vi "Heart Sound TFA.vi"() -> ()   [LabVIEW 2023]
doc: "This example shows the application of the Time Frequency Analysis VIs in heart sound signal processing. \n\nTime frequency analysis has been widely applied in heart sound signal processing. You can use the Time Frequency Spectrogram Express VI to perform different methods for time-frequency representations. The frequency modulation of heart sound signals can be investigated easily in the time-frequency domain.\n\nThis example uses the Time Frequency Spectrogram Express VI to compute the adaptive spectrogram of the heart sound signal and uses the TFA Adaptive Transform VI to detect the modulation parameters of the heart sound signal.\n\n<b>Instructions:</b>\n1) Run this VI.\n2) Observe the <b>Spectrogram of Heart Sound</b> and the values of the detected chirplets in the <b>Chirplet Info</b> to learn the frequency modulation of heart sound."
uses:
  <vilib>/addons/Time Frequency Analysis/typedefs.llb/TFA Data.ctl
  Instance           5 23Saved   Heart Sound TFA .vi
  <vilib>/addons/Time Frequency Analysis/Transform.llb/TFA Adaptive Transform (Waveform).vi
  <vilib>/addons/Time Frequency Analysis/_control.llb/TFA Configure Spectrogram Indicator (Predefined Color Table).vi
  <vilib>/addons/_Advanced Signal Processing/NI_AdvSigProcTFA.lvlib
panel:
  out "aspt-left-top":bool
  out "Chirplet info":T1(array[cluster]) {"chirp rate" format="%#_2p Hz/s"; "frequency" format="%#_2p Hz"; "center" format="%#_2ps"; "standard deviation" format="%#_2ps"; "amplitude" format="%.2p"}
  out "Spectrogram of Heart Sound":dbl[][](graph)
  out "Heart Sound":waveform(dbl)(graph)
  # "Overview: Shows the application of the Time Frequency Analysis VIs in heart sound signal processing.\nRequirements: LabVIEW Full Development System, Advanced Signal Processing Toolkit\nInstructions: \n1. Run this VI.\n2. Observe the Spectrogram of Heart Sound and the values of the detected chirplets in the Chirplet Info to learn the frequency modulation of heart sound."
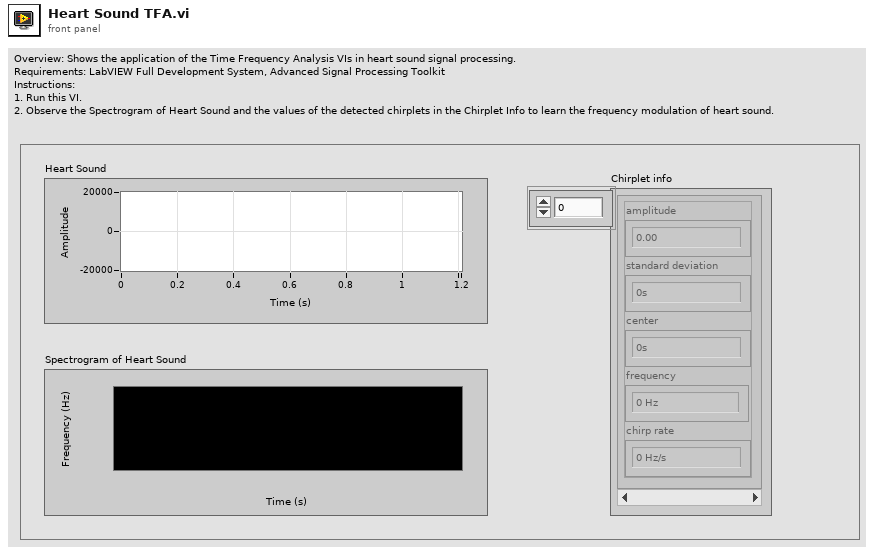
[diagram p1: front panel]
types:
  T1 = cluster{"amplitude":cdb, "standard deviation":dbl, "center":dbl, "frequency":dbl, "chirp rate":dbl}[]
  T2 = typedef "NI_AdvSigProcTFA.lvlib/TFA Data.ctl" = u16
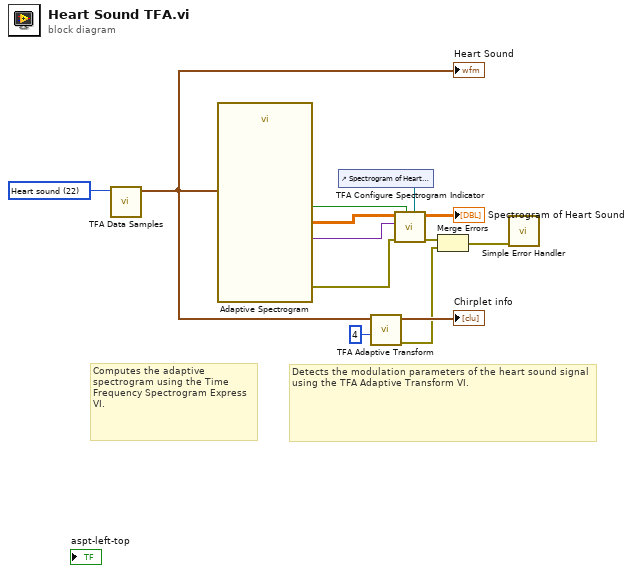
[diagram p0: block diagram]
diagram:
  w5 = T2 22 items=["PC Fan"=0, "Noisy Chirps"=1, "TDR 1"=2, "TDR 2"=3, "Liquefaction"=4, "Liquefaction Free"=5, "Aneurysm"=6, "Bat"=7, "RF"=8, "Two Gaussian"=9, "Three Gaussian"=10, "Chirp"=11, "Gaussian Chirp"=12, "Cross Chirp"=13, "Doppler"=14, "HOP"=15, "TF Sine"=16, "Three Tone"=17, "Four Tone"=23, "Blood Flow Doppler (phase a)"=20, "Blood Flow Doppler (phase b)"=21, "Heart sound"=22, "-"=18, "Random Noise"=19] ("data")
  # "Detects the modulation parameters of the heart sound signal using the TFA Adaptive Transform VI."
  # "Computes the adaptive spectrogram using the Time Frequency Spectrogram Express VI."
  n1 = call <vilib>:"TFA Data Samples.vi"("data"=w5) -> ("signal"=w6:waveform(dbl))  [unwired: 10 out]
  "Heart Sound" <- w6
  n2 = call "Adaptive Spectrogram"("Signal"=w6) -> ("error out"=w4:errorcluster, "Scale Info"=w9:variant, "Spectrogram"=w10:dbl[][], "dB"=w11:bool)  [unwired: 2 in, 5 out]
  n3 = control-ref of="Spectrogram of Heart Sound"() -> (w13:refnum<vi>)
  n4 = call-poly <vilib>:"TFA Adaptive Transform.vi"("number of terms"=4, "signal"=w6) -> ("error out"=w2:errorcluster, "chirplet info"=→"Chirplet info":T1)  [unwired: 1 in, 7 out]
  n5 = call-poly <vilib>:"TFA Configure Spectrogram Indicator.vi"("reference of TF spectrogram indicator"=w13, "dB on? (F)"=w11, "error in (no error)"=w4, "scale info"=w9, "spectrogram"=w10) -> ("error out"=w3:errorcluster, "TF spectrogram indicator"=→"Spectrogram of Heart Sound":dbl[][])  [unwired: 2 in, 3 out]
  n6 = Merge Errors(w3, w2) -> (w1:errorcluster)
  n7 = call <vilib>:"Simple Error Handler.vi"("error in (no error)"=w1) -> ()  [unwired: 4 in, 5 out]
